vi "4. Multi-file configuration system.vi"() -> ()   [LabVIEW 2017]
uses:
  819bf4ab-68c0-4ee7-aa53-d72678bf237b.vi
  5a9b6002-9b4c-44bb-8af0-bdd7d247c2b8.vi
  a0dbf1ed-92c6-47c3-b2e7-8cfb88ce05be.vi
  f65b758a-57a2-4ff6-b8fb-5289b55a65bc.vi
  <userlib>/_NEVSTOP/Communicable State Machine(CSM)/addons/API-String-Arugments-Support/_Support/Concatenate Strings If not Empty_csm.vi
  INI-Static-Variable-Support/_Support/FlagInstance-CSMINIVariable.vi
  5a9b6002-9b4c-44bb-8af0-bdd7d247c2b8.vi/70cf541c-689a-4909-ae73-497058dc5e15.vi
  5a9b6002-9b4c-44bb-8af0-bdd7d247c2b8.vi/8441470c-f7c2-4ba6-a00e-bb382131ed64.vi
  a0dbf1ed-92c6-47c3-b2e7-8cfb88ce05be.vi/70cf541c-689a-4909-ae73-497058dc5e15.vi
  a0dbf1ed-92c6-47c3-b2e7-8cfb88ce05be.vi/8441470c-f7c2-4ba6-a00e-bb382131ed64.vi
  f65b758a-57a2-4ff6-b8fb-5289b55a65bc.vi/99de0c97-112a-4c86-9094-c187659127e1.vi
  <userlib>/_NEVSTOP/Communicable State Machine(CSM)/Utility/Build Error Cluster.vi
  <userlib>/_NEVSTOP/Communicable State Machine(CSM)/_Support/ChangeFlag/ChangeFlag-Read.vi
  5a9b6002-9b4c-44bb-8af0-bdd7d247c2b8.vi/8441470c-f7c2-4ba6-a00e-bb382131ed64.vi/99de0c97-112a-4c86-9094-c187659127e1.vi
  a0dbf1ed-92c6-47c3-b2e7-8cfb88ce05be.vi/8441470c-f7c2-4ba6-a00e-bb382131ed64.vi/99de0c97-112a-4c86-9094-c187659127e1.vi
  <vilib>/Utility/Data Type/Get Type Information.vi
  <userlib>/_NEVSTOP/Communicable State Machine(CSM)/addons/API-String-Arugments-Support/_Support/Data To SingleElementsArray_csm.vi
  <userlib>/_NEVSTOP/Communicable State Machine(CSM)/addons/API-String-Arugments-Support/_Support/Data To API String Arguments.vi
  INI-Static-Variable-Support/_Support/Parse Used Session and Name.vi
  INI-Static-Variable-Support/_Support/INI-FGV(lvlibp).vi
  INI-Static-Variable-Support/_Support/Populate String with INI Variable.vi
  <userlib>/_NEVSTOP/Communicable State Machine(CSM)/addons/API-String-Arugments-Support/_Support/Convert API String Arguments to Data(variant).vi
  <userlib>/_NEVSTOP/Communicable State Machine(CSM)/addons/API-String-Arugments-Support/_Support/SingleElementsArray To Data_csm.vi
  <userlib>/_NEVSTOP/Communicable State Machine(CSM)/_Support/ChangeFlag/ChangeFlagDB.vi
  INI-Static-Variable-Support/_Support/CSM - Read INI String.vi
  INI-Static-Variable-Support/INI-Static-Variable-Support.lvlib
  <vilib>/Instr/_visa.llb/VISA Configure Serial Port (Instr).vi
panel:
  out "Signal":cluster{"k":dbl, "b":dbl}[](array[cluster])=[{"k"=1.2, "b"=0.0}, {"k"=1000.0, "b"=0.0}]
  out "RS232_Device Config 3":T1={"Resource"="com10", "baud rate"=500000, "data bits"=8, "parity"=enum."Odd", "stop bits"=10}
  out "RS232_Device Config 2":T1={"Resource"="com5", "baud rate"=115200, "data bits"=8, "parity"=enum."Odd", "stop bits"=10}
  out "RS232_Device Config":T1={"Resource"="com5", "baud rate"=115200, "data bits"=8, "parity"=enum."Odd", "stop bits"=10}
  # "#CSM-Example overview"
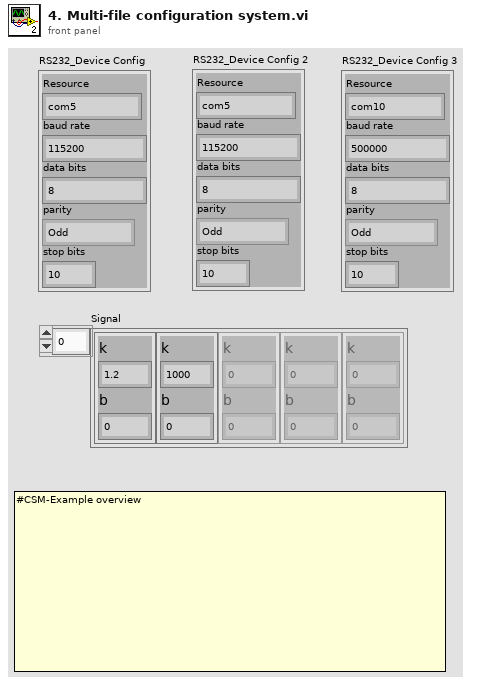
[diagram p1: front panel]
types:
  T1 = cluster{"Resource":string, "baud rate":u32, "data bits":u16, "parity":enum16{"None", "Odd", "Even", "Mark", "Space"}, "stop bits":u16}
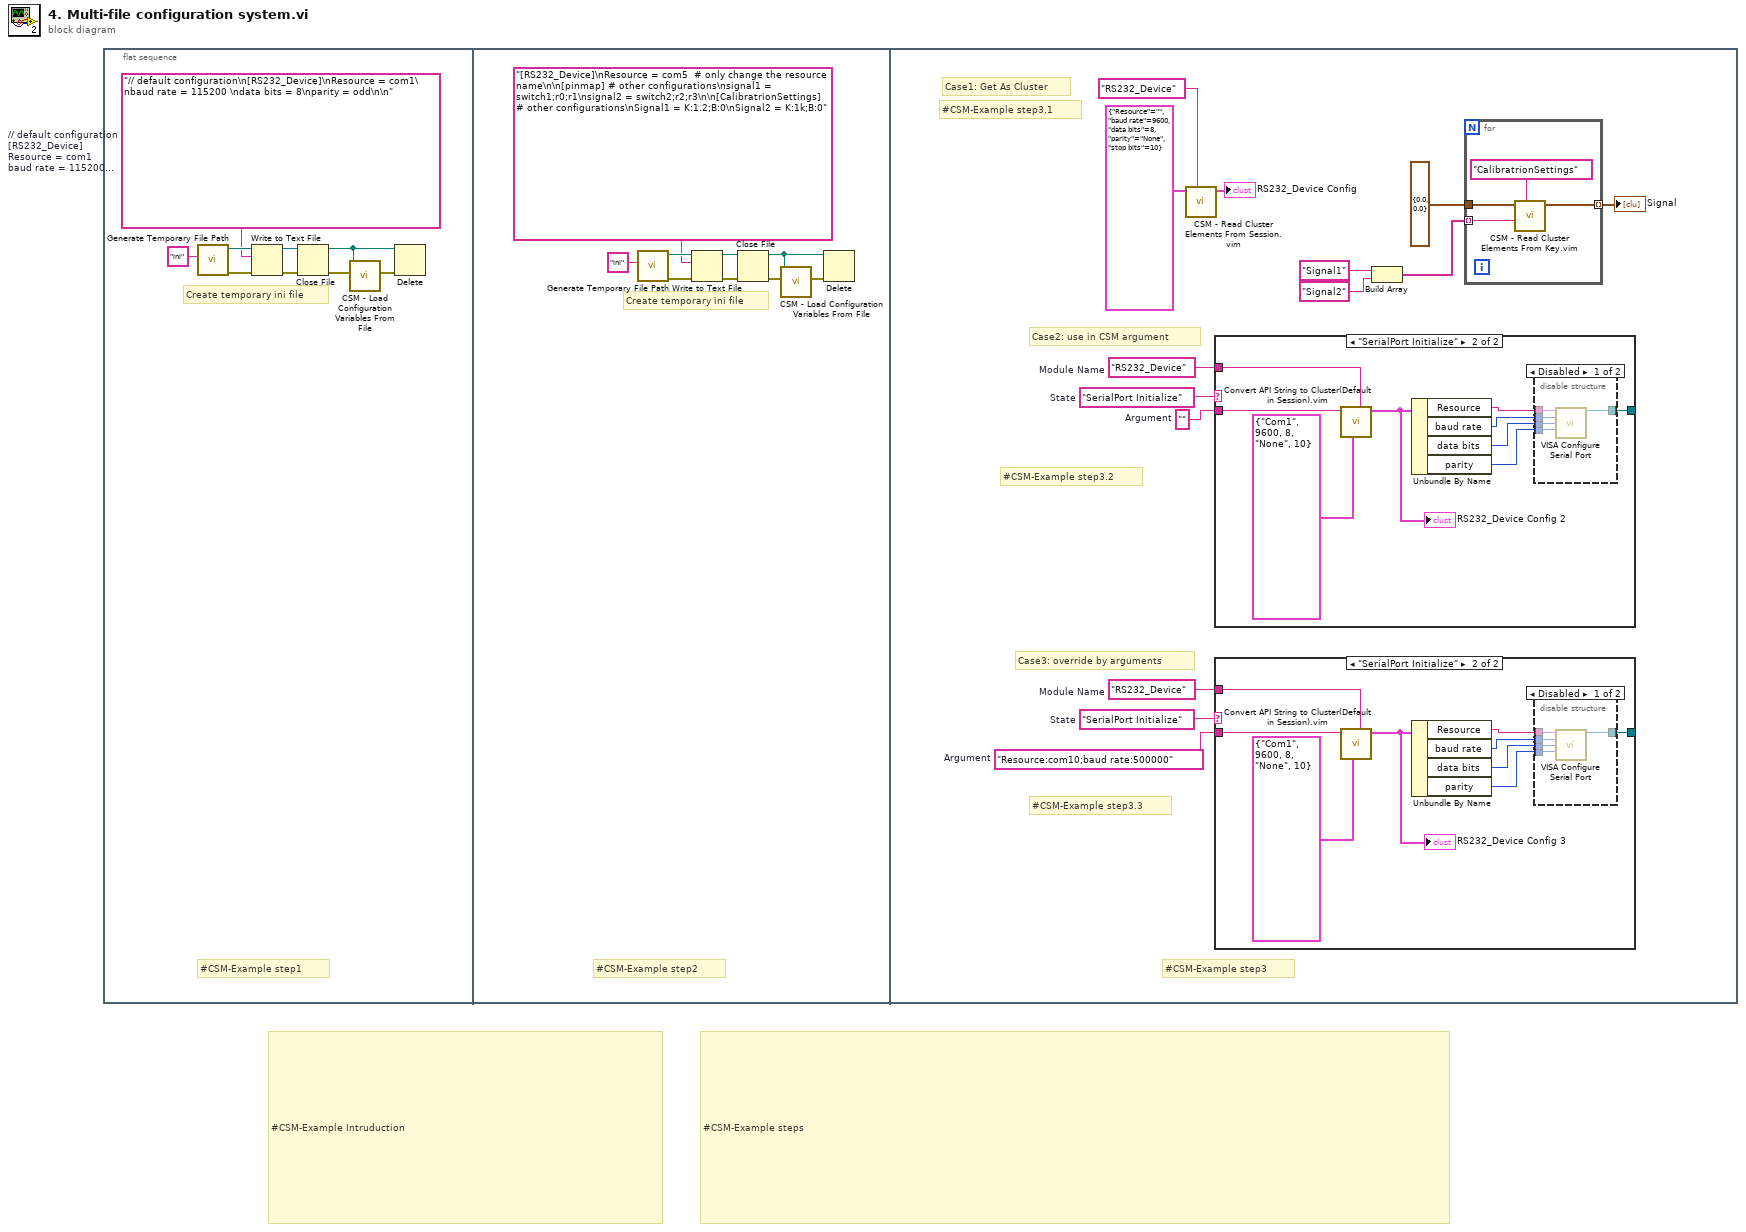
[diagram p0: block diagram]
diagram:
  # "#CSM-Example steps"
  # "#CSM-Example Intruduction"
  n1 = flat-sequence {
    frame #0 {
      w3 = "// default configuration\n[RS232_Device]\nResource = com1\nbaud rate = 115200 \ndata bits = 8\nparity = odd\n\n"  # // default configuration [RS232_Device] Resource = com1 baud rate = 115200  data bits = 8 parity = odd
      # "#CSM-Example step1"
      # "Create temporary ini file"
      n2 = call <vilib>:"Generate Temporary File Path.vi"("Temporary File Extension (tmp)"="ini") -> ("error out"=w9:errorcluster, "Unique Temporary File Path"=w6:path)  [unwired: 9 in]
      n3 = Write to Text File(file (use dialog)=w6, text=w3, error in=w9) -> (refnum out=w5:refnum<file>, error out=w7:errorcluster)  [unwired: 1 in, 1 out]
      n4 = Close File(refnum=w5, error in=w7) -> (path=w1:path, error out=w4:errorcluster)
      n5 = call "CSM - Load Configuration Variables From File.vi"("error in (no error)"=w4, "Configuration Path"=w1) -> ("error out"=w2:errorcluster)  [unwired: 7 in]
      n6 = Delete(path (use dialog)=w1, error in=w2) -> ()  [unwired: 3 in, 3 out]
    }
    frame #1 {
      # "#CSM-Example step2"
      # "Create temporary ini file"
      n7 = call <vilib>:"Generate Temporary File Path.vi"("Temporary File Extension (tmp)"="ini") -> ("error out"=w14:errorcluster, "Unique Temporary File Path"=w16:path)  [unwired: 9 in]
      n8 = Write to Text File(file (use dialog)=w16, text="[RS232_Device]\nResource = com5  # only change the resource name\n\n[pinmap] # other configurations\nsignal1 = switch1;r0;r1\nsignal2 = switch2;r2;r3\n\n[CalibratrionSettings] # other configurations\nSignal1 = K:1.2;B:0\nSignal2 = K:1k;B:0", error in=w14) -> (refnum out=w17:refnum<file>, error out=w15:errorcluster)  [unwired: 1 in, 1 out]
      n9 = Close File(refnum=w17, error in=w15) -> (path=w10:path, error out=w18:errorcluster)
      n10 = call "CSM - Load Configuration Variables From File.vi"("error in (no error)"=w18, "Configuration Path"=w10) -> ("error out"=w11:errorcluster)  [unwired: 7 in]
      n11 = Delete(path (use dialog)=w10, error in=w11) -> ()  [unwired: 3 in, 3 out]
    }
    frame #2 {
      w26 = "Resource:com10;baud rate:500000"  # Argument
      w25 = "RS232_Device"  # Module Name
      w24 = "SerialPort Initialize"  # State
      w27 = ""  # Argument
      w28 = "RS232_Device"  # Module Name
      w29 = "SerialPort Initialize"  # State
      # "#CSM-Example step3.3"
      # "#CSM-Example step3.2"
      # "#CSM-Example step3.1"
      # "#CSM-Example step3"
      # "Case3: override by arguments"
      # "Case1: Get As Cluster"
      # "Case2: use in CSM argument"
      n12 = call "CSM - Read Cluster Elements From Session.vim"("Section Name (\"\" as Default)"="RS232_Device" ("Section Name(\"\" as Default)"), "Cluster"=T1 {"Resource"="", "baud rate"=9600, "data bits"=8, "parity"=enum."None", "stop bits"=10}) -> ("Cluster out"=→"RS232_Device Config":T1)  [unwired: 6 in, 1 out]
      n13 = case shown="\"SerialPort Initialize\"" w29 {
        tunnel: w28 -> [_ w57]
        tunnel: w27 -> [_ w59]
        tunnel: [_ w51] -> _
        frame Default {
        }
        frame "SerialPort Initialize" {
          n14 = call "Convert API String to Cluster(Default in Session).vim"("Section Name(\"\" as Default)"=w57, "Type"=T1 {"Resource"="Com1", "baud rate"=9600, "data bits"=8, "parity"=enum."None", "stop bits"=10}, "API String"=w59) -> ("Data"=w56:T1)  [unwired: 7 in, 1 out]
          "RS232_Device Config 2" <- w56
          n15 = Unbundle By Name(w56) -> ("Resource"=w55:string, "baud rate"=w52:u32, "data bits"=w53:u16, "parity"=w54:enum16{"None", "Odd", "Even", "Mark", "Space"})
          n16 = disable-structure shown="Disabled" {
            disable-tunnel: w55 -> [w64 _]
            disable-tunnel: w54 -> [w63 _]
            disable-tunnel: w53 -> [w62 _]
            disable-tunnel: w52 -> [w61 _]
            disable-tunnel: [w60 _] -> w51
            frame Disabled {
              n17 = call-poly "VISA Configure Serial Port"("VISA resource name"=w64, "baud rate (9600)"=w61, "data bits (8)"=w62, "parity (0:none)"=w63) -> ("VISA resource name out"=w60:refnum<visa-resource-name>)  [unwired: 10 in, 1 out]
            }
            frame Enabled {
            }
          }
        }
      }
      n18 = case shown="\"SerialPort Initialize\"" w24 {
        tunnel: w25 -> [_ w43]
        tunnel: w26 -> [_ w45]
        tunnel: [_ w37] -> _
        frame Default {
        }
        frame "SerialPort Initialize" {
          n19 = call "Convert API String to Cluster(Default in Session).vim"("Section Name(\"\" as Default)"=w43, "Type"=T1 {"Resource"="Com1", "baud rate"=9600, "data bits"=8, "parity"=enum."None", "stop bits"=10}, "API String"=w45) -> ("Data"=w42:T1)  [unwired: 7 in, 1 out]
          "RS232_Device Config 3" <- w42
          n20 = Unbundle By Name(w42) -> ("Resource"=w41:string, "baud rate"=w38:u32, "data bits"=w39:u16, "parity"=w40:enum16{"None", "Odd", "Even", "Mark", "Space"})
          n21 = disable-structure shown="Disabled" {
            disable-tunnel: w41 -> [w50 _]
            disable-tunnel: w40 -> [w49 _]
            disable-tunnel: w39 -> [w48 _]
            disable-tunnel: w38 -> [w47 _]
            disable-tunnel: [w46 _] -> w37
            frame Disabled {
              n22 = call-poly "VISA Configure Serial Port"("VISA resource name"=w50, "baud rate (9600)"=w47, "data bits (8)"=w48, "parity (0:none)"=w49) -> ("VISA resource name out"=w46:refnum<visa-resource-name>)  [unwired: 10 in, 1 out]
            }
            frame Enabled {
            }
          }
        }
      }
      n23 = Build Array("Signal1" ("Key"), "Signal2" ("Key")) -> (w20:string[])
      n24 = for {
        tunnel: w20 -> [w33] mode=indexing
        tunnel: cluster{"k":dbl, "b":dbl} {"k"=0.0, "b"=0.0} -> [w36]
        tunnel: [w34] -> w21 mode=indexing
        n25 = call "CSM - Read Cluster Elements From Key.vim"("Section Name (\"\" as Default)"="CalibratrionSettings" ("Section Name(\"\" as Default)"), "Key"=w33, "Cluster"=w36) -> ("Cluster out"=w34:cluster{"k":dbl, "b":dbl})  [unwired: 4 in, 2 out]
      }
      "Signal" <- w21
    }
  }
